vi "Marker Opposite Visible Read.vi"(8 "error in (no error)":errorcluster, 11 "3D Plot.lvclass in":refnum<class "3D Plot.lvclass">) -> (0 "error out":errorcluster, 1 "Label Opposite Visible?":bool, 3 "3D Plot.lvclass out":refnum<class "3D Plot.lvclass">)   [LabVIEW 2020, in "3D Plot.lvclass"]
uses:
  3D Plot.lvclass
  3D Plot.lvclass/3D Plot.ctl
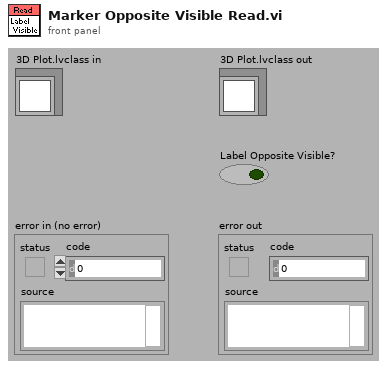
[diagram p1: front panel]
types:
  T1 = cluster{"Show Normal X Label":bool, "Show Normal Y Label":bool, "Show Normal Z Label":bool, "Show Opposite X Label":bool, "Show Opposite Y Label":bool, "Show Opposite Z Label":bool}
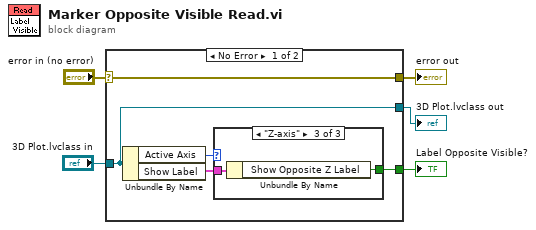
[diagram p0: block diagram]
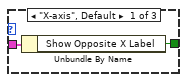
[diagram p2: hidden frame]
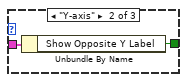
[diagram p3: hidden frame]
diagram:
  n1 = case shown="No Error" "error in (no error)" {
    selector: "error in (no error)" -> [w6 w17]
    tunnel: [w10 _] -> w5
    tunnel: "3D Plot.lvclass in" -> [w7 w18]
    tunnel: [w7 w18] -> w3
    tunnel: [w6 w17] -> w2
    frame No Error {
      n2 = Unbundle By Name(w7) -> ("Active Axis"=w8:enum16{"X-axis", "Y-axis", "Z-axis"}, "Show Label"=w9:T1)
      n3 = case shown="\"Z-axis\"" w8 {
        tunnel: w9 -> [w11 w14 w16]
        tunnel: [w12 w13 w15] -> w10
        frame "X-axis", Default {
          n4 = Unbundle By Name(w11) -> ("Show Opposite X Label"=w12:bool)
        }
        frame "Y-axis" {
          n5 = Unbundle By Name(w14) -> ("Show Opposite Y Label"=w13:bool)
        }
        frame "Z-axis" {
          n6 = Unbundle By Name(w16) -> ("Show Opposite Z Label"=w15:bool)
        }
      }
    }
    frame Error {
    }
  }
  "error out" <- w2
  "Label Opposite Visible?" <- w5
  "3D Plot.lvclass out" <- w3
